vi "demod_limiter.vi"(6 "Reset":bool, 10 "Config":T2={"I/O"={"Format"={"Rate"=4, "Bits"=32, "Channels"=2}, "card #"=1, "# buffers"=96000}, "High rate STFT"={"Win param"=101.5, "Window type"=61, "Win order"=2, "DFT size"=64, "Channels"=[7], "Oversample"=64}, "Low rate STFT"={"Win param"=120.0, "Window type"=61, "Win order"=8, "DFT size"=64, "Channels"=[7], "Oversample"=64}, "Filtering"={"Hum"={"Frequency"=0.0, "Tc"=0.0, "Limit"=101.5, "FFT filter"=FALSE, "Detrend mode"=enum."Robust linear", "Enable"=FALSE}, "Kalman"={"Process noise"=101.5, "Measure noise"=101.5, "Unlock m noise"=101.5, "Mode"=enum."FFT"}, "Distortion"={"LF cut"=101.5, "Tc"=3.0, "Limit"=101.5, "FFT filter"=FALSE, "Detrend mode"=enum."Robust linear", "Enable"=FALSE}, "Lowpass"={"Frequency"=0.0, "Order"=0, "Enable"=FALSE}, "Impulse"={"Win order"=102, "Locked limit"=101.5, "Locked count"=102, "Threshold Tc"=101.5, "Thresh sigmas"=101.5, "Thresh min"=101.5, "After"=0, "Detrend"=FALSE, "Enable"=FALSE}}} {"Filtering"."Impulse"."Thresh min" format="%#_3p"; "Filtering"."Impulse"."Threshold Tc" format="%#_3p"; "Filtering"."Impulse"."Locked limit" format="%#_3p"; "Filtering"."Impulse"."Thresh sigmas" format="%#_3p"; "Filtering"."Lowpass"."Frequency" format="%#_4p"; "Filtering"."Distortion"."Limit" format="%#_3p"; "Filtering"."Distortion"."LF cut" format="%#_3p"; "Filtering"."Kalman"."Unlock m noise" format="%#_3p"; "Filtering"."Kalman"."Measure noise" format="%#_3p"; "Filtering"."Kalman"."Process noise" format="%#_3p"; "Filtering"."Hum"."Limit" format="%#_3p"; "Filtering"."Hum"."Frequency" format="%#_4p"; "Low rate STFT"."Oversample" min=1 step=1; "Low rate STFT"."Channels" min=0 step=1; "Low rate STFT"."DFT size" min=1 step=1; "Low rate STFT"."Window type" items=["Rectangle"=0, "Hanning"=1, "Hamming"=2, "Blackman-Harris"=3, "Exact Blackman"=4, "Blackman"=5, "Flat Top"=6, "4 Term B-Harris "=7, "7 Term B-Harris"=8, "Low Sidelobe"=9, "Blackman Nuttall"=11, "Triangle"=30, "Bartlett-Hanning"=31, "Bohman"=32, "Parzen"=33, "Welch"=34, "Kaiser"=60, "Dolph-Chebyshev"=61, "Gaussian"=62]; "High rate STFT"."Oversample" min=1 step=1; "High rate STFT"."Channels" min=0 step=1; "High rate STFT"."DFT size" min=1 step=1; "High rate STFT"."Window type" items=["Rectangle"=0, "Hanning"=1, "Hamming"=2, "Blackman-Harris"=3, "Exact Blackman"=4, "Blackman"=5, "Flat Top"=6, "4 Term B-Harris "=7, "7 Term B-Harris"=8, "Low Sidelobe"=9, "Blackman Nuttall"=11, "Triangle"=30, "Bartlett-Hanning"=31, "Bohman"=32, "Parzen"=33, "Welch"=34, "Kaiser"=60, "Dolph-Chebyshev"=61, "Gaussian"=62]}, 11 "Residue in":dbl[](array[numeric])) -> (0 "Impulse":bool, 1 "Unlocked":bool, 2 "Residue w/ trend":dbl[](array[numeric]), 3 "Residue out":dbl[](array[numeric]))   [LabVIEW 2014]
uses:
  ilemt_config.ctl
  io_config.ctl
  stft_params.ctl
  <vilib>/Analysis/4window.llb/windowTd.ctl
  filter_params.ctl
  detrend_mode.ctl
  modulation_info.ctl
  <vilib>/Analysis/6fits.llb/Curve Fitting Criteria.ctl
  <vilib>/Analysis/5stat.llb/RMS (DBL).vi
  <vilib>/Analysis/NI_AALPro.lvlib
panel:
  out "Trend":dbl(graph)
  out "RMS":dbl(graph)
  in  "Modulation info":T1={"Fs full"=0.0, "Fs high"=0.0, "Fs low"=0.0, "Read size"=5000, "FFT size low"=5000, "df low"=5000.0, "High carriers"=[], "Low carriers"=[], "Hi channels at low"=[7]} {"Hi channels at low" min=0 step=1; "Low carriers" format="%#_6p"; "High carriers" format="%#_6p"}
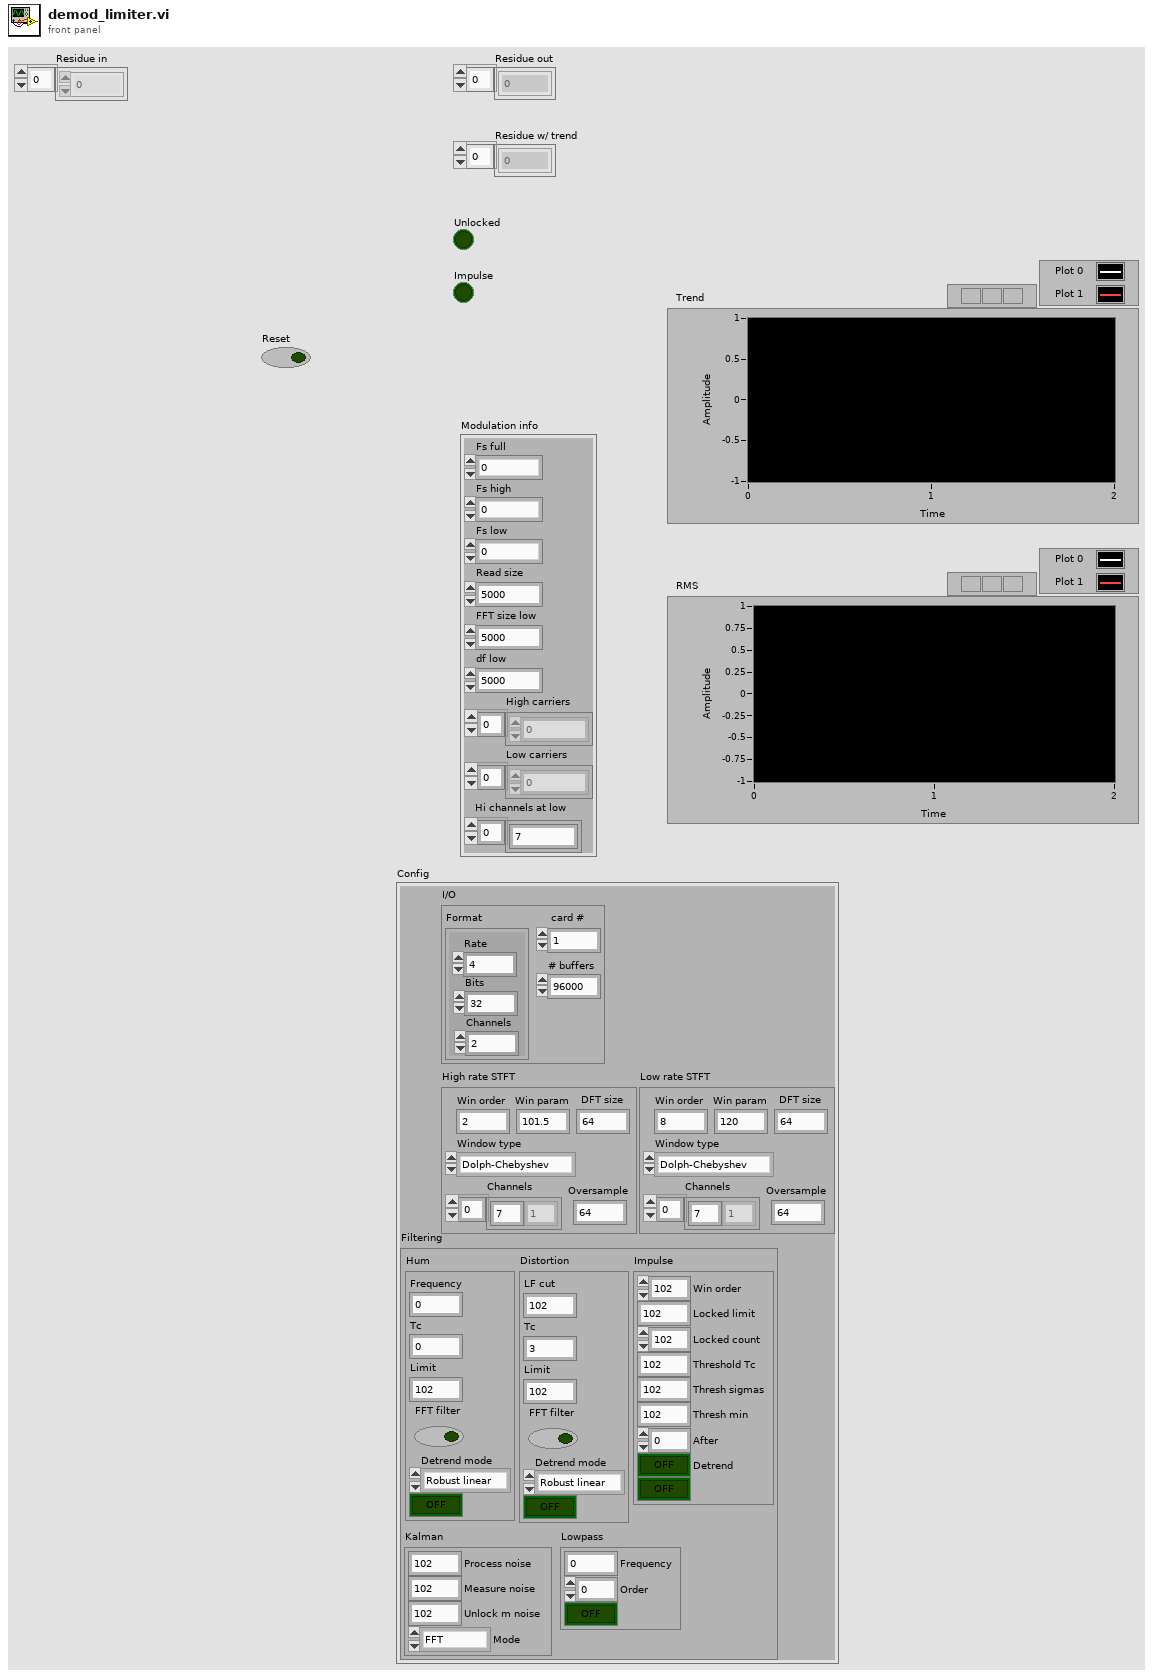
[diagram p1: front panel]
types:
  T1 = typedef "modulation_info.ctl" = cluster{"Fs full":dbl, "Fs high":dbl, "Fs low":dbl, "Read size":i32, "FFT size low":i32, "df low":dbl, "High carriers":dbl[], "Low carriers":dbl[], "Hi channels at low":i32[]}
  T2 = typedef "ilemt_config.ctl" = cluster{"I/O":T3, "High rate STFT":T4, "Low rate STFT":T4, "Filtering":T6}
  T3 = typedef "io_config.ctl" = cluster{"Format":cluster{"Rate":i32, "Bits":i32, "Channels":u32}, "card #":u32, "# buffers":i32}
  T4 = typedef "stft_params.ctl" = cluster{"Win param":dbl, "Window type":T5, "Win order":i32, "DFT size":i32, "Channels":i32[], "Oversample":i32}
  T5 = typedef "NI_AALPro.lvlib/windowTd.ctl" = u32
  T6 = typedef "filter_params.ctl" = cluster{"Hum":cluster{"Frequency":dbl, "Tc":dbl, "Limit":dbl, "FFT filter":bool, "Detrend mode":T7, "Enable":bool}, "Kalman":cluster{"Process noise":dbl, "Measure noise":dbl, "Unlock m noise":dbl, "Mode":enum16{"FFT", "KF demod"}}, "Distortion":cluster{"LF cut":dbl, "Tc":dbl, "Limit":dbl, "FFT filter":bool, "Detrend mode":T7, "Enable":bool}, "Lowpass":cluster{"Frequency":dbl, "Order":i32, "Enable":bool}, "Impulse":cluster{"Win order":i32, "Locked limit":dbl, "Locked count":i32, "Threshold Tc":dbl, "Thresh sigmas":dbl, "Thresh min":dbl, "After":i32, "Detrend":bool, "Enable":bool}}
  T7 = typedef "detrend_mode.ctl" = enum16{"Zero mean", "Linear", "Robust linear"}
  T8 = typedef "NI_AALPro.lvlib/Curve Fitting Criteria.ctl" = u16
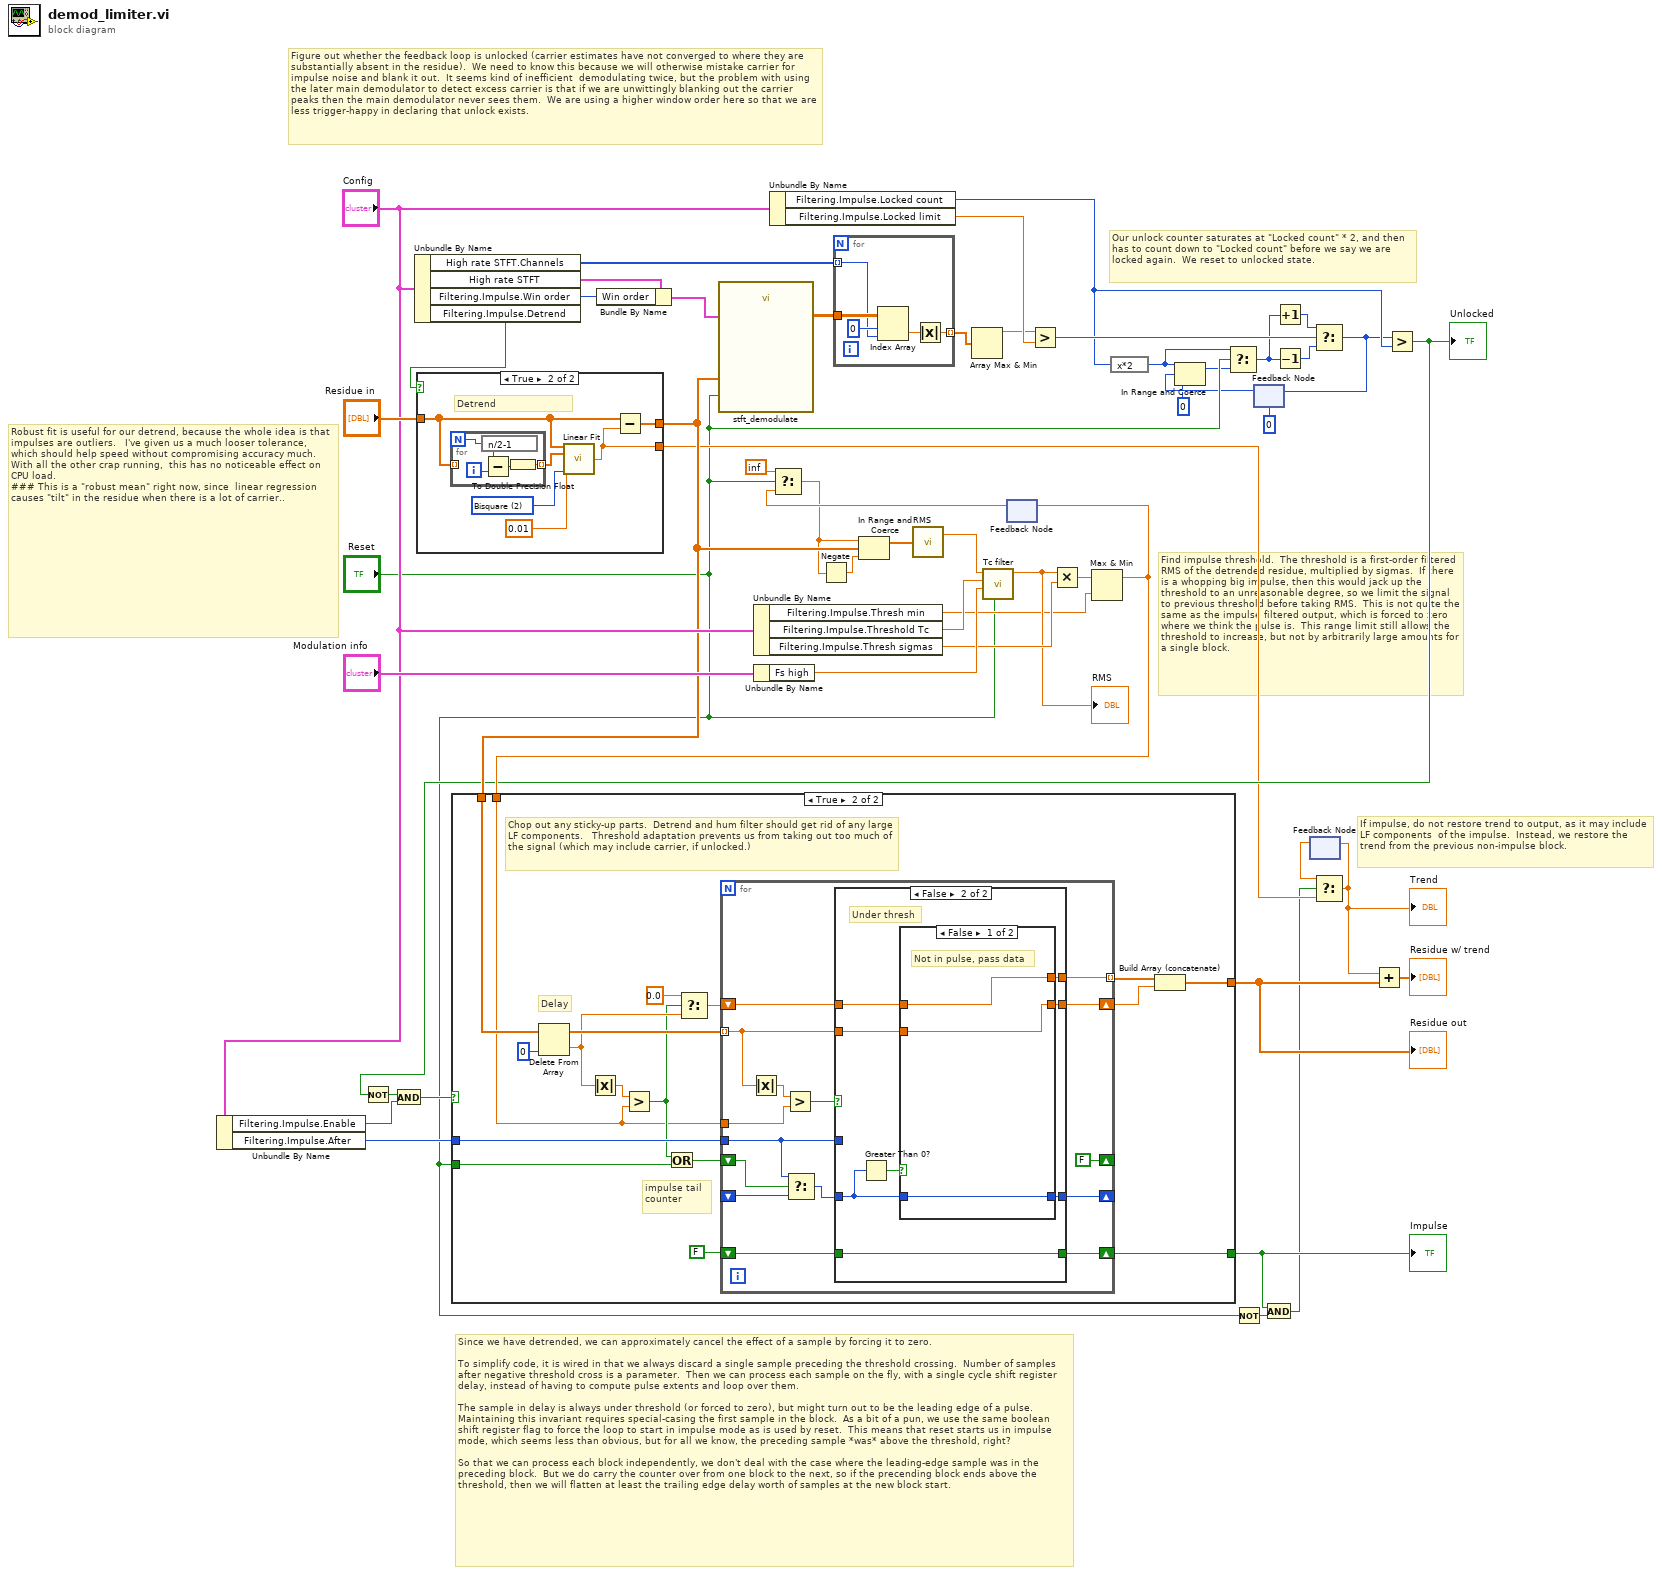
[diagram p0: block diagram]
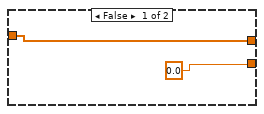
[diagram p2: hidden frame]
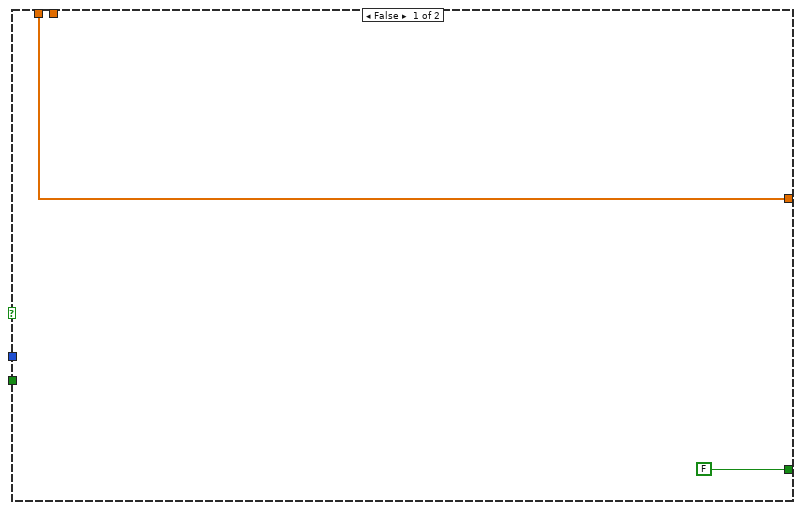
[diagram p3: hidden frame]
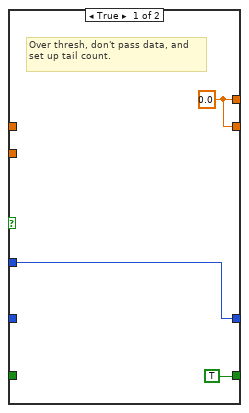
[diagram p4: hidden frame]
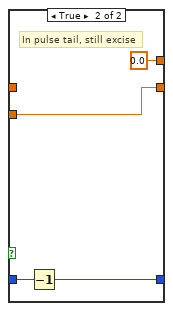
[diagram p5: hidden frame]
diagram:
  # "Figure out whether the feedback loop is unlocked (carrier estimates have not converged to where they are substantially absent in the residue).  We need to know this because we will otherwise mistake carrier for impulse noise and blank it out.  It seems kind of inefficient  demodulating twice, but the problem with using the later main demodulator to detect excess carrier is that if we are unwittingly blanking out the carrier peaks then the main demodulator never sees them.  We are using a higher window order here so that we are less trigger-happy in declaring that unlock exists."
  # "Our unlock counter saturates at \"Locked count\" * 2, and then has to count down to \"Locked count\" before we say we are locked again.  We reset to unlocked state."
  # "If impulse, do not restore trend to output, as it may include LF components  of the impulse.  Instead, we restore the trend from the previous non-impulse block."
  # "Find impulse threshold.  The threshold is a first-order filtered RMS of the detrended residue, multiplied by sigmas.  If there is a whopping big impulse, then this would jack up the threshold to an unreasonable degree, so we limit the signal to previous threshold before taking RMS.  This is not quite the same as the impulse filtered output, which is forced to zero where we think the pulse is.  This range limit still allows the threshold to increase, but not by arbitrarily large amounts for a single block."
  # "Robust fit is useful for our detrend, because the whole idea is that impulses are outliers.   I've given us a much looser tolerance, which should help speed without compromising accuracy much.  With all the other crap running,  this has no noticeable effect on CPU load.\n### This is a \"robust mean\" right now, since  linear regression causes \"tilt\" in the residue when there is a lot of carrier.."
  # "Since we have detrended, we can approximately cancel the effect of a sample by forcing it to zero. \n\nTo simplify code, it is wired in that we always discard a single sample preceding the threshold crossing.  Number of samples after negative threshold cross is a parameter.  Then we can process each sample on the fly, with a single cycle shift register delay, instead of having to compute pulse extents and loop over them.  \n\nThe sample in delay is always under threshold (or forced to zero), but might turn out to be the leading edge of a pulse.  Maintaining this invariant requires special-casing the first sample in the block.  As a bit of a pun, we use the same boolean shift register flag to force the loop to start in impulse mode as is used by reset.  This means that reset starts us in impulse mode, which seems less than obvious, but for all we know, the preceding sample *was* above the threshold, right?\n\nSo that we can process each block independently, we don't deal with the case where the leading-edge sample was in the preceding block.  But we do carry the counter over from one block to the next, so if the precending block ends above the threshold, then we will flatten at least the trailing edge delay worth of samples at the new block start."
  n1 = Unbundle By Name("Config") -> ("Filtering.Impulse.Enable"=w20:bool, "Filtering.Impulse.After"=w45:i32)
  n2 = Unbundle By Name("Config") -> ("High rate STFT.Channels"=w3:i32[], "High rate STFT"=w49:T4, "Filtering.Impulse.Win order"=w47:i32, "Filtering.Impulse.Detrend"=w44:bool)
  n3 = case shown="True" w44 {
    tunnel: "Residue in" -> [w53 w59]
    tunnel: [w53 w57] -> w31
    tunnel: [0.0 ("t") w54] -> w18
    frame False {
    }
    frame True {
      w56 = T8 2 items=["Least Square", "Least Absolute Residual", "Bisquare"] ("method")
      # "Detrend"
      n4 = for {
        N -> [w63]
        tunnel: w59 -> [_] mode=indexing
        tunnel: [w64] -> w58 mode=indexing
        i -> [w62]
        n5 = expression code="n/2-1"(w63) -> (w60:i32)
        n6 = Subtract(x=w60, y=w62) -> (x-y=w61:i32)
        n7 = To Double Precision Float(number=w61) -> (double precision float=w64:dbl)
      }
      n8 = call <vilib>:"Linear Fit.vi"("Y"=w59, "X"=w58, "tolerance"=0.01, "method"=w56) -> ("intercept"=w54:dbl)  [unwired: 7 in, 4 out]
      n9 = Subtract(x=w59, y=w54) -> (x-y=w57:dbl[])
    }
  }
  n10 = Bundle By Name(cluster=w49, "Win order"=w47) -> (w48:T4)
  n11 = call "stft_demodulate.vi"("STFT params"=w48, "Reset"="Reset", "X"=w31) -> ("STFT"=w50:cdb[][])  [unwired: 6 in, 2 out]
  n12 = Unbundle By Name("Config") -> ("Filtering.Impulse.Thresh min"=w32:dbl, "Filtering.Impulse.Threshold Tc"=w37:dbl, "Filtering.Impulse.Thresh sigmas"=w36:dbl)
  n13 = Unbundle By Name("Modulation info") -> ("Fs high"=w39:dbl)
  n14 = Unbundle By Name("Config") -> ("Filtering.Impulse.Locked count"=w6:i32, "Filtering.Impulse.Locked limit"=w46:dbl)
  n15 = for {
    tunnel: w50 -> [w69]
    tunnel: [w67] -> w2 mode=indexing
    tunnel: w3 -> [w65] mode=indexing
    n16 = Index Array(array=w69, index (row)=0 ("disabled index (row)"), index (col)=w65) -> (element=w66:cdb)
    n17 = Absolute Value(x=w66) -> (abs(x)=w67:dbl)
  }
  n18 = Array Max & Min(array=w2) -> (max value=w1:dbl)  [unwired: 3 out]
  n19 = feedback #1() -> (w25:dbl)  [unwired: 1 in]
  n20 = Select(t=inf, s="Reset", f=w25) -> (s? t:f=w24:dbl)
  n21 = Negate(x=w24) -> (-x=w29:dbl)
  n22 = In Range and Coerce(upper limit=w24, x=w31, lower limit=w29) -> (coerced(x)=w30:dbl[])  [unwired: 1 out]
  n23 = call-poly <vilib>:"RMS.vi"("X"=w30) -> ("rms value"=w28:dbl)  [unwired: 1 out]
  n24 = call "Tc filter.vi"("Reset"="Reset", "Fs"=w39, "Tc"=w37, "Input"=w28) -> ("Output"=w34:dbl)  [unwired: 7 in]
  "RMS" <- w34
  n25 = Greater?(x=w1, y=w46) -> (0:w42:bool)
  n26 = Multiply(x=w34, y=w36) -> (x*y=w33:dbl)
  n27 = Max & Min(x=w33, y=w32) -> (max(x,y)=w27:dbl)  [unwired: 1 out]
  n28 = feedback-in #1(w27) -> ()
  n29 = expression code="x*2"(w6) -> (w4:i32)
  n30 = Not(x="Reset") -> (.not. x?=w17:bool)
  n31 = feedback #2(0 ("disabled index (row)")) -> (w9:i32)
  n32 = In Range and Coerce(upper limit=w4, x=w9, lower limit=0) -> (coerced(x)=w8:i32)  [unwired: 1 out]
  n33 = Select(t=w4, s="Reset", f=w8) -> (s? t:f=w11:i32)
  n34 = Increment(x=w11) -> (x+1=w41:i32)
  n35 = Decrement(x=w11) -> (x-1=w13:i32)
  n36 = feedback #3() -> (w19:dbl)  [unwired: 1 in]
  n37 = Select(t=w41, s=w42, f=w13) -> (s? t:f=w5:i32)
  n38 = feedback-in #2(w5) -> ()
  n39 = Greater?(x=w5, y=w6) -> (0:w22:bool)
  "Unlocked" <- w22
  n40 = Not(x=w22) -> (.not. x?=w23:bool)
  n41 = And(x=w23, y=w20) -> (x .and. y?=w21:bool)
  n42 = case shown="True" w21 {
    tunnel: w31 -> [w71 w87]
    tunnel: "Reset" -> [_ w80]
    tunnel: w45 -> [_ w88]
    tunnel: [w71 w82] -> w35
    tunnel: [FALSE w73] -> w16
    tunnel: w27 -> [_ w72]
    frame False {
    }
    frame True {
      # "Delay"
      # "impulse tail counter"
      # "Chop out any sticky-up parts.  Detrend and hum filter should get rid of any large LF components.   Threshold adaptation prevents us from taking out too much of the signal (which may include carrier, if unlocked.)"
      n43 = Delete From Array(array=w87, index=0) -> (deleted portion=w78:dbl, array with subset deleted=w85:dbl[])  [unwired: 1 in]
      n44 = Absolute Value(x=w78) -> (abs(x)=w81:dbl)
      n45 = Greater?(x=w81, y=w72) -> (0:w76:bool)
      n46 = Or(x=w76, y=w80) -> (x .or. y?=w79:bool)
      n47 = Select(t=0.0, s=w76, f=w78) -> (s? t:f=w77:dbl)
      n48 = for {
        tunnel: w85 -> [w96] mode=indexing
        shift-right: [w100] -> _
        shift-left: _ -> [w95]
        tunnel: w72 -> [w103]
        tunnel: w88 -> [w93]
        shift-right: [w97] -> w83
        shift-left: w77 -> [w99]
        tunnel: [w98] -> w84 mode=indexing
        shift-right: [FALSE] -> _
        shift-left: w79 -> [w94]
        shift-right: [w89] -> w73
        shift-left: FALSE -> [w90]
        n49 = Absolute Value(x=w96) -> (abs(x)=w102:dbl)
        n50 = Greater?(x=w102, y=w103) -> (0:w101:bool)
        n51 = Select(t=w93, s=w94, f=w95) -> (s? t:f=w92:i32)
        n52 = case shown="False" w101 {
          tunnel: w92 -> [_ w113]
          tunnel: w93 -> [w106 _]
          tunnel: [w106 w112] -> w100
          tunnel: w99 -> [_ w111]
          tunnel: [w105 w110] -> w98
          tunnel: [w105 w109] -> w97
          tunnel: w96 -> [_ w108]
          tunnel: w90 -> [_ w107]
          tunnel: [TRUE w107] -> w89
          frame True {
            w105 = 0.0
            # "Over thresh, don't pass data, and set up tail count."
          }
          frame False {
            # "Under thresh"
            n53 = Greater Than 0?(x=w113) -> (x > 0?=w114:bool)
            n54 = case shown="False" w114 {
              tunnel: w113 -> [w115 w121]
              tunnel: [w115 w120] -> w112
              tunnel: w111 -> [w117 _]
              tunnel: [w117 0.0] -> w110
              tunnel: [w116 w119] -> w109
              tunnel: w108 -> [w116 w119]
              frame False {
                # "Not in pulse, pass data"
              }
              frame True {
                # "In pulse tail, still excise"
                n55 = Decrement(x=w121) -> (x-1=w120:i32)
              }
            }
          }
        }
      }
      n56 = Build Array (concatenate)(w84, w83) -> (w82:dbl[])
    }
  }
  "Residue out" <- w35
  "Impulse" <- w16
  n57 = And(x=w16, y=w17) -> (x .and. y?=w15:bool)
  n58 = Select(t=w19, s=w15, f=w18) -> (s? t:f=w14:dbl)
  "Trend" <- w14
  n59 = feedback-in #3(w14) -> ()
  n60 = Add(x=w14, y=w35) -> (x+y=→"Residue w/ trend":dbl[])
